vi "Documentation.vi"   [LabVIEW 2019, in "Inst.KH7008.lvlib" / "Inst.Krohn-Hite-7008.lvclass"]
uses:
  Inst.Krohn-Hite-7008.lvclass
  <vilib>/JKI/JKI SMO/SMO/SMO.lvclass
  Typedefs/Inst.Krohn-Hite-7008.getAll--Cluster.ctl
  Typedefs/Inst.Krohn-Hite-7008.device--Cluster.ctl
  Inst UI.Krohn-Hite-7008/Inst UI.Krohn-Hite-7008.lvclass
  Inst UI.Krohn-Hite-7008/Inst UI.Krohn-Hite-7008.UI--Cluster.ctl
  <userlib>/LevyLab/Instrument Framework/Instrument UI/Instrument UI.lvclass
  C:/Program Files (x86)/National Instruments/LabVIEW 2019/user.lib/LevyLab/Instrument Framework/Instrument Types/Amplifier/Instrument.Amplifier.lvclass
  C:/Program Files (x86)/National Instruments/LabVIEW 2019/user.lib/LevyLab/Instrument Framework/Instrument/Instrument.lvclass
  C:/Program Files (x86)/National Instruments/LabVIEW 2019/vi.lib/JKI/JKI SMO/SMO/SMO.lvclass
  Typedefs/Inst.Krohn-Hite-7008.Commands--Enum.ctl
  <userlib>/LevyLab/Instrument Framework/Instrument/Instrument.lvclass
  KH7008/typedefs/Input--Enum.ctl
  KH7008/KH7008.lvlib
  KH7008/typedefs/couple--Enum.ctl
  KH7008/typedefs/shunt--enum.ctl
  KH7008/typedefs/Filter--Enum.ctl
  KH7008/typedefs/gain--enum.ctl
  KH7008/typedefs/channel--numeric.ctl
  KH7008/typedefs/channelProperties--Cluster.ctl
  KH7008/typedefs/allChannelProperties--Array.ctl
  Typedefs/setAllChannelsRequest--Cluster.ctl
  C:/Program Files (x86)/National Instruments/LabVIEW 2019/user.lib/LevyLab/Instrument Framework/Instrument UI/Instrument UI.lvclass
  C:/Program Files (x86)/National Instruments/LabVIEW 2019/vi.lib/JKI/JKI SMO/SMO.UI/SMO.UI.lvclass
  <vilib>/JKI/JKI SMO/SMO.UI/SMO.UI.lvclass
  <userlib>/LevyLab/RemoteControl/RemoteControl/RemoteControl.lvclass
  <userlib>/LevyLab/Instrument Framework/Instrument/API/Instrument.sendMessageToProcess (string).vi
types:
  T1 = typedef "Inst.KH7008.lvlib/Inst.Krohn-Hite-7008.lvclass/Inst.Krohn-Hite-7008.device--Cluster.ctl" = cluster{"model":string, "device_id":string}
  T2 = typedef "Inst.KH7008.lvlib/Inst.Krohn-Hite-7008.lvclass/Inst.Krohn-Hite-7008.getAll--Cluster.ctl" = cluster{"allChannelProperties":T3}
  T3 = typedef "KH7008.lvlib/allChannelProperties--Array.ctl" = T4[]
  T4 = typedef "KH7008.lvlib/channelProperties--Cluster.ctl" = cluster{"channel":T5, "gain":T6, "input":T7, "shunt":T8, "couple":T9, "filter":T10}
  T5 = typedef "KH7008.lvlib/channel--numeric.ctl" = u16
  T6 = typedef "KH7008.lvlib/gain--enum.ctl" = enum16{"1", "10", "100", "1000"}
  T7 = typedef "KH7008.lvlib/Input--Enum.ctl" = enum16{"OFF", "SE+", "SE-", "DIFF"}
  T8 = typedef "KH7008.lvlib/shunt--enum.ctl" = enum16{"Open", "50", "500", "5k", "50k", "10M"}
  T9 = typedef "KH7008.lvlib/couple--Enum.ctl" = enum16{"AC", "DC"}
  T10 = typedef "KH7008.lvlib/Filter--Enum.ctl" = enum16{"OFF", "ON"}
  T11 = typedef "Inst.KH7008.lvlib/Inst.Krohn-Hite-7008.lvclass/Inst.Krohn-Hite-7008.Commands--Enum.ctl" = enum16{"getChannel", "getAllChannels", "setChannel", "setAllChannels"}
  T12 = typedef "Inst.KH7008.lvlib/Inst UI.Krohn-Hite-7008.lvclass/Inst UI.Krohn-Hite-7008.UI--Cluster.ctl" = cluster{"setAllChannelsRequest":T13}
  T13 = typedef "Inst.KH7008.lvlib/Inst.Krohn-Hite-7008.lvclass/setAllChannelsRequest--Cluster.ctl" = cluster{"allChannelProperties":T3}
  T14 = typedef "Instrument.lvlib/Instrument.lvclass/PublicEvents--Cluster.ctl" = cluster{"MessageFromProcess":refnum<user-event>}
  T15 = typedef "Instrument.lvlib/Instrument.lvclass/PrivateEvents--Cluster.ctl" = cluster{"MessageToProcess":refnum<user-event>, "LogData":refnum<user-event>, "LogDataMultiline":refnum<user-event>}
  T16 = typedef "Inst.KH7008.lvlib/Inst.Krohn-Hite-7008.lvclass/PublicEvents--Cluster.ctl" = cluster{"MessageFromProcess":refnum<user-event>}
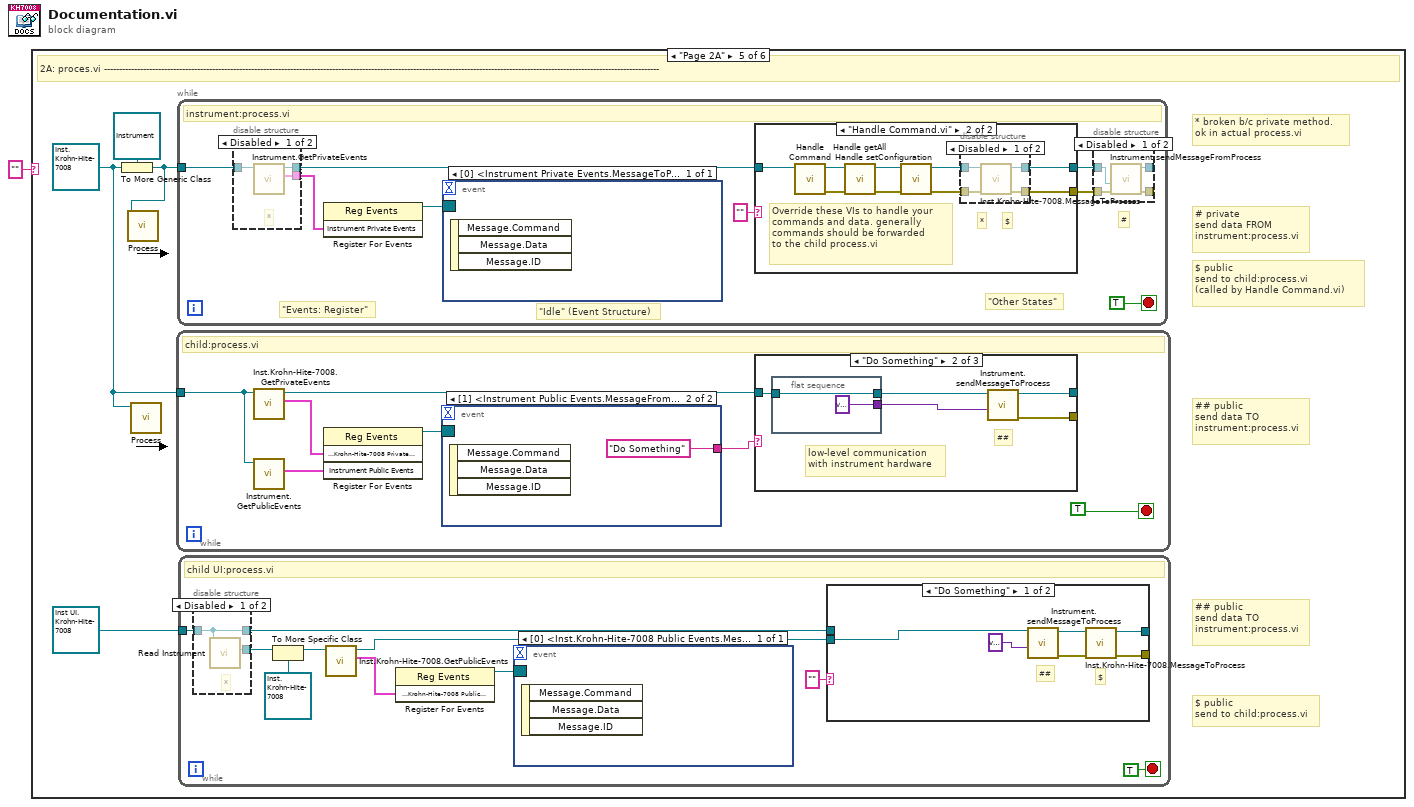
[diagram p0: block diagram]
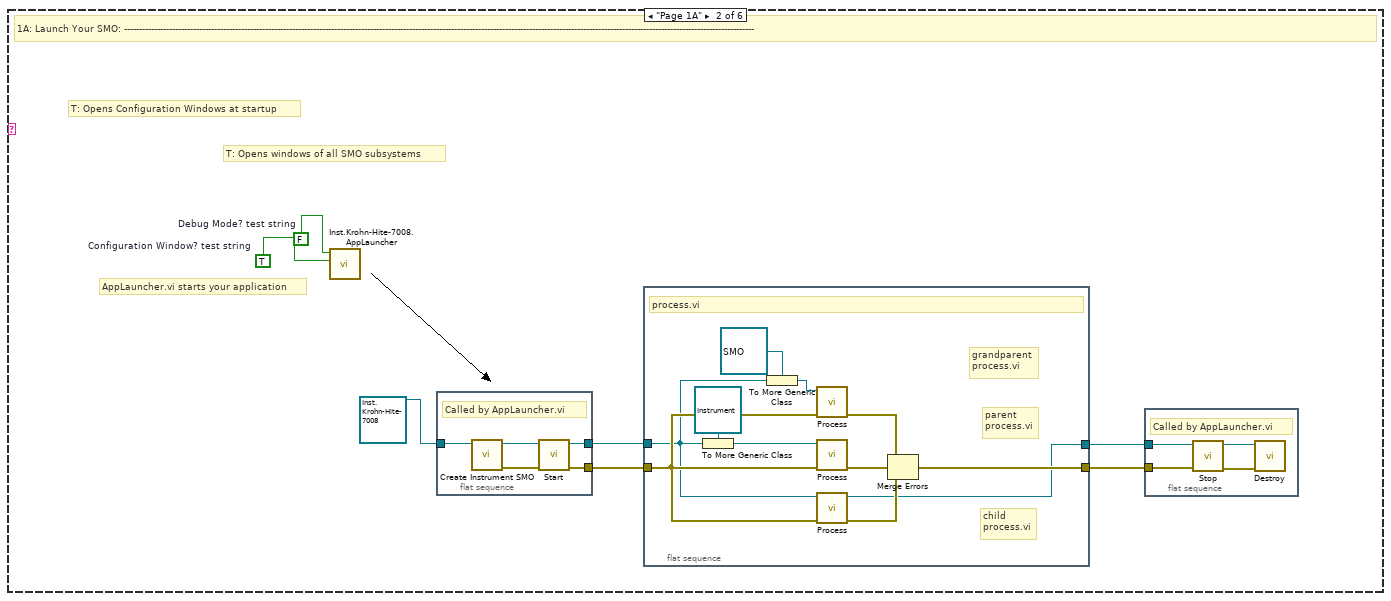
[diagram p3: hidden frame]
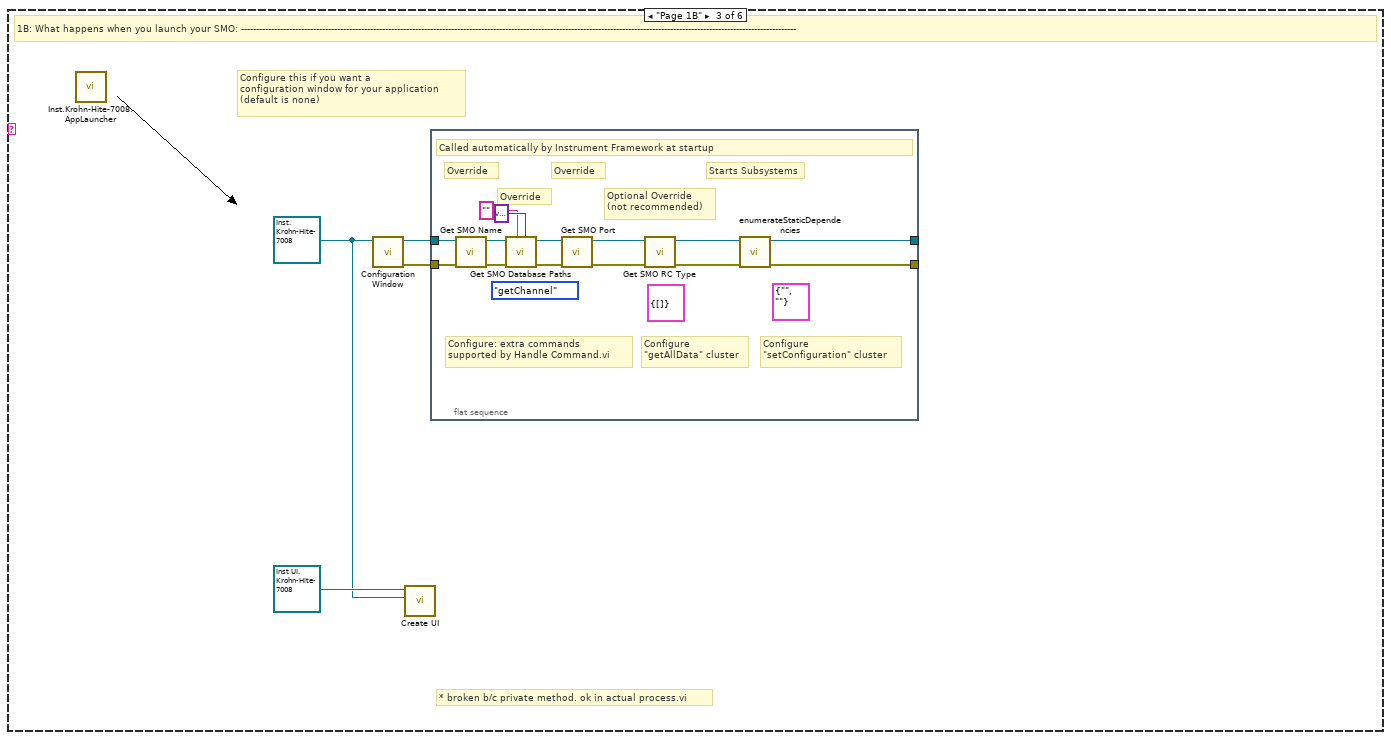
[diagram p4: hidden frame]
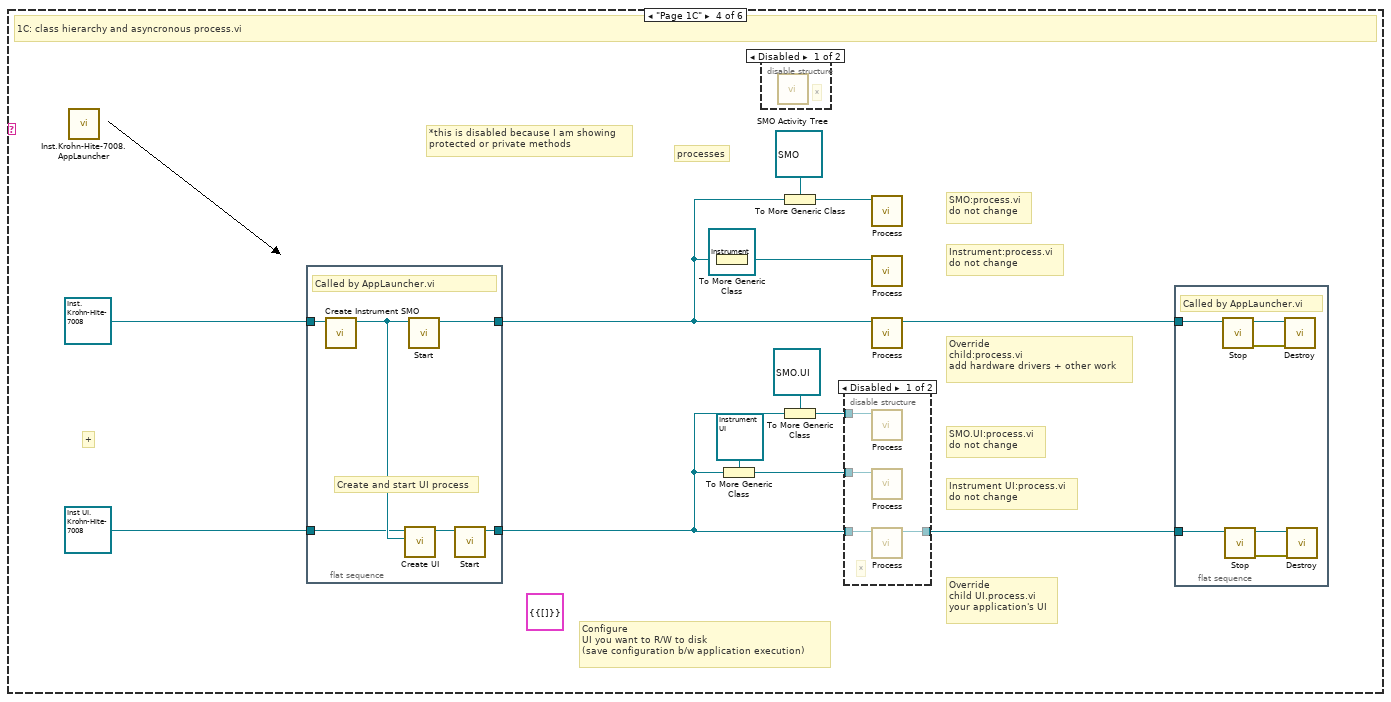
[diagram p5: hidden frame]
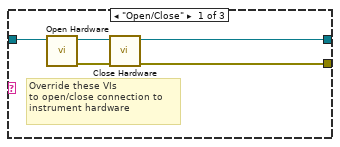
[diagram p10: hidden frame]
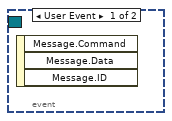
[diagram p12: hidden frame]
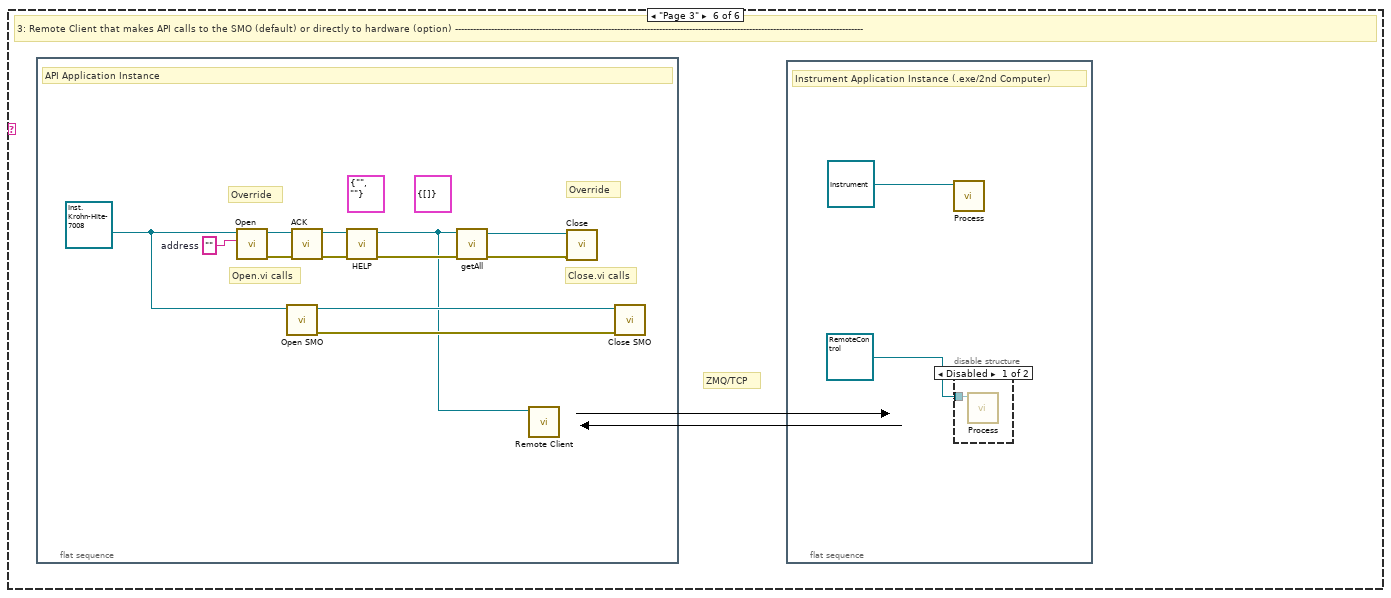
[diagram p17: hidden frame]
diagram:
  n1 = case shown="\"Page 2A\"" "" {
    frame Default {
    }
    frame "Page 1A" {
      w7 = TRUE  # Configuration Window? test string
      w8 = FALSE  # Debug Mode? test string
      # "AppLauncher.vi starts your application"
      # "T: Opens windows of all SMO subsystems"
      # "T: Opens Configuration Windows at startup"
      # "1A: Launch Your SMO: ------------------------------------------------------------------------------------------------------------------------------------------------------------------------------------------------------------------"
      n2 = call "Inst.Krohn-Hite-7008.AppLauncher.vi"("Config Window"=w7, "Debug Mode"=w8) -> ()  [unwired: 9 in, 1 out]
      n3 = flat-sequence {
        tunnel: [w26] -> w3
        tunnel: [w25] -> w5
        tunnel: refnum<class "Inst.Krohn-Hite-7008.lvclass"> refnum ("Instrument.Template.lvclass") -> [w24]
        frame #0 {
          # "Called by AppLauncher.vi"
          n4 = call <userlib>:"Create Instrument SMO.vi"("Instrument in"=w24) -> ("error out"=w27:errorcluster, "Instrument out"=w28:refnum<class "Inst.Krohn-Hite-7008.lvclass">)  [unwired: 9 in]
          n5 = call <vilib>:"Start.vi"("error in (no error)"=w27, "SMO"=w28) -> ("error out"=w25:errorcluster, "SMO out"=w26:refnum<class "Inst.Krohn-Hite-7008.lvclass">)  [unwired: 8 in]
        }
      }
      n6 = flat-sequence {
        tunnel: [w19] -> w6
        tunnel: w5 -> [w17]
        tunnel: [w11] -> w4
        tunnel: w3 -> [w10]
        frame #0 {
          # "child\nprocess.vi"
          # "grandparent\nprocess.vi"
          # "parent\nprocess.vi"
          # "process.vi"
          n7 = To More Generic Class(target class=refnum<class "Instrument.lvclass"> refnum ("Instrument"), reference=w10) -> (generic class reference=w16:refnum<class "Instrument.lvclass">)
          n8 = To More Generic Class(target class=refnum<class "SMO.lvclass"> refnum ("SMO"), reference=w10) -> (generic class reference=w18:refnum<class "SMO.lvclass">)
          n9 = call-dynamic "Process.vi"("error in"=w17, "SMO"=w18) -> ("error out"=w12:errorcluster)  [unwired: 8 in, 1 out]
          n10 = call-dynamic "Process.vi"("error in"=w17, "Instrument"=w16) -> ("error out"=w14:errorcluster)  [unwired: 8 in, 1 out]
          n11 = call-dynamic "Process.vi"("error in"=w17, "Inst.Krohn-Hite-7008"=w10) -> ("error out"=w13:errorcluster, "Inst.Krohn-Hite-7008 out"=w11:refnum<class "Inst.Krohn-Hite-7008.lvclass">)  [unwired: 8 in]
          n12 = Merge Errors(w12, w14, w13) -> (w19:errorcluster)
        }
      }
      n13 = flat-sequence {
        tunnel: w4 -> [w21]
        tunnel: w6 -> [w20]
        frame #0 {
          # "Called by AppLauncher.vi"
          n14 = call <vilib>:"Stop.vi"("error in (no error)"=w20, "SMO"=w21) -> ("error out"=w23:errorcluster, "SMO out"=w22:refnum<class "Inst.Krohn-Hite-7008.lvclass">)  [unwired: 8 in]
          n15 = call <vilib>:"Destroy.vi"("error in (no error)"=w23, "SMO"=w22) -> ()  [unwired: 9 in, 1 out]
        }
      }
    }
    frame "Page 1B" {
      w29 = refnum<class "Inst.Krohn-Hite-7008.lvclass"> refnum ("Instrument.Template.lvclass")
      # "* broken b/c private method. ok in actual process.vi"
      # "Configure this if you want a\nconfiguration window for your application\n(default is none)"
      # "1B: What happens when you launch your SMO: -----------------------------------------------------------------------------------------------------------------------------------------------------------------------------------------"
      n16 = call "Inst.Krohn-Hite-7008.AppLauncher.vi"() -> ()  [unwired: 11 in, 1 out]
      n17 = call-dynamic "Configuration Window.vi"("Inst.Krohn-Hite-7008 in"=w29) -> ("error out"=w31:errorcluster, "Inst.Krohn-Hite-7008 out"=w32:refnum<class "Inst.Krohn-Hite-7008.lvclass">)  [unwired: 9 in]
      n18 = call <userlib>:"Create UI.vi"("Instrument in"=w29, "Instrument UI"=refnum<class "Inst UI.Krohn-Hite-7008.lvclass"> refnum ("Instrument UI.Template.lvclass")) -> ()  [unwired: 8 in, 2 out]
      n19 = flat-sequence {
        tunnel: w32 -> [w42]
        tunnel: w31 -> [w37]
        tunnel: [w36] -> _
        tunnel: [w35] -> _
        frame #0 {
          (unwired) T1 {"model"="", "device_id"=""} ("Configuration")
          (unwired) T2 {"allChannelProperties"=[]} ("getAll")
          (unwired) Inst.Krohn-Hite-7008.Commands--Enum."getChannel" ("Commands")
          # "Configure\n\"setConfiguration\" cluster"
          # "Configure\n\"getAllData\" cluster"
          # "Configure: extra commands\nsupported by Handle Command.vi"
          # "Starts Subsystems"
          # "Override"
          # "Override"
          # "Override"
          # "Optional Override\n(not recommended)"
          # "Called automatically by Instrument Framework at startup"
          n20 = call-dynamic "Get SMO Name.vi"("error in (no error)"=w37, "Inst.Krohn-Hite-7008 in"=w42) -> ("error out"=w40:errorcluster, "Inst.Krohn-Hite-7008 out"=w41:refnum<class "Inst.Krohn-Hite-7008.lvclass">)  [unwired: 7 in, 1 out]
          n21 = call-dynamic "Get SMO Database Paths.vi"("getAll Cluster"=variant, "Paths"="" ("Default Paths"), "error in (no error)"=w40, "Inst.Krohn-Hite-7008 in"=w41) -> ("error out"=w38:errorcluster, "Inst.Krohn-Hite-7008 out"=w39:refnum<class "Inst.Krohn-Hite-7008.lvclass">)  [unwired: 5 in, 1 out]
          n22 = call-dynamic "Get SMO Port.vi"("error in (no error)"=w38, "Inst.Krohn-Hite-7008Instrument in"=w39) -> ("error out"=w43:errorcluster, "Inst.Krohn-Hite-7008Instrument out"=w44:refnum<class "Inst.Krohn-Hite-7008.lvclass">)  [unwired: 7 in, 1 out]
          n23 = call-dynamic "Get SMO RC Type.vi"("error in (no error)"=w43, "Instrument in"=w44) -> ("error out"=w45:errorcluster, "Instrument out"=w46:refnum<class "Inst.Krohn-Hite-7008.lvclass">)  [unwired: 7 in, 1 out]
          n24 = call-dynamic "enumerateStaticDependencies.vi"("error in (no error)"=w45, "Instrument"=w46) -> ("error out"=w36:errorcluster, "Instrument out"=w35:refnum<class "Inst.Krohn-Hite-7008.lvclass">)  [unwired: 7 in, 1 out]
        }
      }
    }
    frame "Page 1C" {
      (unwired) T12 {"setAllChannelsRequest"={"allChannelProperties"=[]}} ("UI")
      # "processes"
      # "SMO.UI:process.vi\ndo not change"
      # "Instrument UI:process.vi\ndo not change"
      # "Override\nchild:process.vi\nadd hardware drivers + other work"
      # "SMO:process.vi\ndo not change"
      # "Instrument:process.vi\ndo not change"
      # "*this is disabled because I am showing\nprotected or private methods"
      # "Configure\nUI you want to R/W to disk\n(save configuration b/w application execution)"
      # "Override\nchild UI.process.vi\nyour application's UI"
      # "+"
      # "1C: class hierarchy and asyncronous process.vi"
      n25 = call "Inst.Krohn-Hite-7008.AppLauncher.vi"() -> ()  [unwired: 11 in, 1 out]
      n26 = flat-sequence {
        tunnel: [w76] -> w59
        tunnel: refnum<class "Inst.Krohn-Hite-7008.lvclass"> refnum ("Instrument.Template.lvclass") -> [w75]
        tunnel: refnum<class "Inst UI.Krohn-Hite-7008.lvclass"> refnum ("Instrument UI.Template.lvclass") -> [w73]
        tunnel: [w71] -> w57
        frame #0 {
          # "Create and start UI process"
          # "Called by AppLauncher.vi"
          n27 = call <userlib>:"Create Instrument SMO.vi"("Instrument in"=w75) -> ("Instrument out"=w74:refnum<class "Inst.Krohn-Hite-7008.lvclass">)  [unwired: 9 in, 1 out]
          n28 = call <userlib>:"Create UI.vi"("Instrument in"=w74, "Instrument UI"=w73) -> ("Instrument UI out"=w72:refnum<class "Inst UI.Krohn-Hite-7008.lvclass">)  [unwired: 8 in, 1 out]
          n29 = call <vilib>:"Start.vi"("SMO"=w74) -> ("SMO out"=w76:refnum<class "Inst.Krohn-Hite-7008.lvclass">)  [unwired: 9 in, 1 out]
          n30 = call <vilib>:"Start.vi"("SMO"=w72) -> ("SMO out"=w71:refnum<class "Inst UI.Krohn-Hite-7008.lvclass">)  [unwired: 9 in, 1 out]
        }
      }
      n31 = To More Generic Class(target class=refnum<class "Instrument.lvclass"> refnum ("Instrument"), reference=w59) -> (generic class reference=w54:refnum<class "Instrument.lvclass">)
      n32 = To More Generic Class(target class=refnum<class "Instrument UI.lvclass"> refnum ("Instrument UI"), reference=w57) -> (generic class reference=w50:refnum<class "Instrument UI.lvclass">)
      n33 = disable-structure shown="Disabled" {
        frame Disabled {
          # "*"
          n34 = call <vilib>:"SMO Activity Tree.vi"() -> ()  [unwired: 12 in]
        }
        frame Enabled {
        }
      }
      n35 = To More Generic Class(target class=refnum<class "SMO.lvclass"> refnum ("SMO"), reference=w59) -> (generic class reference=w55:refnum<class "SMO.lvclass">)
      n36 = To More Generic Class(target class=refnum<class "SMO.UI.lvclass"> refnum ("SMO.UI"), reference=w57) -> (generic class reference=w48:refnum<class "SMO.UI.lvclass">)
      n37 = disable-structure shown="Disabled" {
        disable-tunnel: w57 -> [w64 _]
        disable-tunnel: [w63 _] -> w56
        disable-tunnel: w50 -> [w62 _]
        disable-tunnel: w48 -> [w61 _]
        frame Disabled {
          # "*"
          n38 = call-dynamic "Process.vi"("SMO.UI"=w61) -> ()  [unwired: 9 in, 2 out]
          n39 = call-dynamic "Process.vi"("Instrument UI in"=w62) -> ()  [unwired: 9 in, 2 out]
          n40 = call-dynamic "Process.vi"("Inst UI.Krohn-Hite-7008"=w64) -> ("Inst UI.Krohn-Hite-7008 out"=w63:refnum<class "Inst UI.Krohn-Hite-7008.lvclass">)  [unwired: 9 in, 1 out]
        }
        frame Enabled {
        }
      }
      n41 = call-dynamic "Process.vi"("SMO"=w55) -> ()  [unwired: 9 in, 2 out]
      n42 = call-dynamic "Process.vi"("Instrument"=w54) -> ()  [unwired: 9 in, 2 out]
      n43 = call-dynamic "Process.vi"("Inst.Krohn-Hite-7008"=w59) -> ("Inst.Krohn-Hite-7008 out"=w60:refnum<class "Inst.Krohn-Hite-7008.lvclass">)  [unwired: 9 in, 1 out]
      n44 = flat-sequence {
        tunnel: w60 -> [w68]
        tunnel: w56 -> [w66]
        frame #0 {
          # "Called by AppLauncher.vi"
          n45 = call <vilib>:"Stop.vi"("SMO"=w68) -> ("error out"=w70:errorcluster, "SMO out"=w69:refnum<class "Inst.Krohn-Hite-7008.lvclass">)  [unwired: 9 in]
          n46 = call <vilib>:"Stop.vi"("SMO"=w66) -> ("error out"=w67:errorcluster, "SMO out"=w65:refnum<class "Inst UI.Krohn-Hite-7008.lvclass">)  [unwired: 9 in]
          n47 = call <vilib>:"Destroy.vi"("error in (no error)"=w70, "SMO"=w69) -> ()  [unwired: 9 in, 1 out]
          n48 = call <vilib>:"Destroy.vi"("error in (no error)"=w67, "SMO"=w65) -> ()  [unwired: 9 in, 1 out]
        }
      }
    }
    frame "Page 2A" {
      w77 = refnum<class "Inst.Krohn-Hite-7008.lvclass"> refnum ("Instrument.Template.lvclass")
      # "## public\nsend data TO\ninstrument:process.vi"
      # "$ public\nsend to child:process.vi"
      # "## public\nsend data TO\ninstrument:process.vi"
      # "$ public\nsend to child:process.vi\n(called by Handle Command.vi)"
      # "# private\nsend data FROM\ninstrument:process.vi"
      # "* broken b/c private method.\nok in actual process.vi"
      # "2A: proces.vi -----------------------------------------------------------------------------------------------------------------------------------------------------------------------------------------"
      n49 = To More Generic Class(target class=refnum<class "Instrument.lvclass"> refnum ("Instrument"), reference=w77) -> (generic class reference=w78:refnum<class "Instrument.lvclass">)
      n50 = call-dynamic "Process.vi"("Instrument"=w78) -> ()  [unwired: 9 in, 2 out]
      n51 = call-dynamic "Process.vi"("Inst.Krohn-Hite-7008"=w77) -> ()  [unwired: 9 in, 2 out]
      n52 = while {
        tunnel: w77 -> [w103]
        stop <- TRUE stop-if-true
        # "child:process.vi"
        n53 = call "Inst.Krohn-Hite-7008.GetPrivateEvents.vi"("Inst.Krohn-Hite-7008 in"=w103) -> ("Inst.Krohn-Hite-7008 Private Events"=w107:cluster{"MessageToProcess":refnum<user-event>}, "Inst.Krohn-Hite-7008 out"=w105:refnum<class "Inst.Krohn-Hite-7008.lvclass">)  [unwired: 8 in, 1 out]
        n54 = call <userlib>:"Instrument.GetPublicEvents.vi"("Instrument"=w103) -> ("Instrument Public Events"=w104:T14)  [unwired: 8 in, 2 out]
        n55 = register-events(w107, w104) -> (reference out=w106:refnum<event-registration>)  [unwired: 2 in, 1 out]
        n56 = event shown="[1] <Instrument Public Events.MessageFromProcess>: User Event" {
          selector: w106 -> [_ _]
          dyn-events: _ -> [_ _]
          timeout: _ -> [_ _]
          tunnel: [_ "Do Something"] -> w101
          event User Event {
            n57 = event-data() -> ()  [unwired: 1 in, 3 out]
          }
          event User Event {
            n58 = event-data() -> ()  [unwired: 1 in, 3 out]
          }
        }
        n59 = case shown="\"Do Something\"" w101 {
          tunnel: w105 -> [w110 w115 w120]
          tunnel: [w109 w117 w120] -> _
          tunnel: [w108 w116 _] -> _
          frame "Open/Close" {
            # "Override these VIs\nto open/close connection to\ninstrument hardware"
            n60 = call-dynamic "Open Hardware.vi"("Inst.Krohn-Hite-7008 in"=w110) -> ("error out"=w112:errorcluster, "Inst.Krohn-Hite-7008 out"=w111:refnum<class "Inst.Krohn-Hite-7008.lvclass">)  [unwired: 9 in]
            n61 = call-dynamic "Close Hardware.vi"("error in (no error)"=w112, "Inst.Krohn-Hite-7008 in"=w111) -> ("error out"=w108:errorcluster, "Inst.Krohn-Hite-7008 out"=w109:refnum<class "Inst.Krohn-Hite-7008.lvclass">)  [unwired: 8 in]
          }
          frame "Do Something" {
            # "##"
            # "low-level communication\nwith instrument hardware"
            n62 = flat-sequence {
              tunnel: w115 -> [w119]
              tunnel: [w119] -> w114
              tunnel: [variant ("Data")] -> w113
              frame #0 {
              }
            }
            n63 = call-poly <userlib>:"Instrument.sendMessageToProcess.vi"("Data"=w113, "Instrument"=w114) -> ("error out"=w116:errorcluster, "Instrument out"=w117:refnum<class "Inst.Krohn-Hite-7008.lvclass">)  [unwired: 8 in]
          }
          frame Default {
          }
        }
      }
      n64 = while {
        tunnel: w78 -> [w128]
        stop <- TRUE stop-if-true
        # "#"
        # "\"Other States\""
        # "\"Idle\" (Event Structure)"
        # "\"Events: Register\""
        # "instrument:process.vi"
        n65 = disable-structure shown="Disabled" {
          disable-tunnel: w128 -> [w152 w153]
          disable-tunnel: [w151 w153] -> w127
          disable-tunnel: [w150 _] -> w126
          frame Disabled {
            # "*"
            n66 = call <userlib>:"Instrument.GetPrivateEvents.vi"("Instrument"=w152) -> ("Instrument Private Events"=w150:T15, "Instrument out"=w151:refnum<class "Instrument.lvclass">)  [unwired: 8 in, 1 out]
          }
          frame Enabled {
          }
        }
        n67 = register-events(w126) -> (reference out=w125:refnum<event-registration>)  [unwired: 2 in, 1 out]
        n68 = event shown="[0] <Instrument Private Events.MessageToProcess>: User Event" {
          selector: w125 -> [_]
          dyn-events: _ -> [_]
          timeout: _ -> [_]
          event User Event {
            n69 = event-data() -> ()  [unwired: 1 in, 3 out]
          }
        }
        n70 = case shown="\"Handle Command.vi\"" "" {
          tunnel: w127 -> [w134 w143]
          tunnel: [w134 w137] -> w124
          tunnel: [_ w136] -> w123
          frame Default {
          }
          frame "Handle Command.vi" {
            # "*"
            # "$"
            # "Override these VIs to handle your\ncommands and data. generally \ncommands should be forwarded\nto the child process.vi"
            n71 = call-dynamic "Handle Command.vi"("Instrument in"=w143) -> ("error out"=w139:errorcluster, "Instrument out"=w142:refnum<class "Instrument.lvclass">)  [unwired: 7 in, 2 out]
            n72 = call-dynamic "Handle getAll.vi"("error in (no error)"=w139, "Instrument in"=w142) -> ("error out"=w140:errorcluster, "Instrument out"=w141:refnum<class "Instrument.lvclass">)  [unwired: 7 in, 1 out]
            n73 = call-dynamic "Handle setConfiguration.vi"("error in (no error)"=w140, "Instrument in"=w141) -> ("error out"=w135:errorcluster, "Instrument out"=w138:refnum<class "Instrument.lvclass">)  [unwired: 8 in]
            n74 = disable-structure shown="Disabled" {
              disable-tunnel: w138 -> [w147 w149]
              disable-tunnel: [w146 w149] -> w137
              disable-tunnel: [w145 w148] -> w136
              disable-tunnel: w135 -> [w144 w148]
              frame Disabled {
                n75 = call "Inst.Krohn-Hite-7008.MessageToProcess.vi"("error in (no error)"=w144, "Inst.Krohn-Hite-7008 in"=w147) -> ("error out"=w145:errorcluster, "Inst.Krohn-Hite-7008 out"=w146:refnum<class "Inst.Krohn-Hite-7008.lvclass">)  [unwired: 8 in]
              }
              frame Enabled {
              }
            }
          }
        }
        n76 = disable-structure shown="Disabled" {
          disable-tunnel: w124 -> [w133 _]
          disable-tunnel: w123 -> [w132 _]
          disable-tunnel: [w131 _] -> _
          disable-tunnel: [w130 _] -> _
          frame Disabled {
            n77 = call <userlib>:"Instrument.sendMessageFromProcess.vi"("error in (no error)"=w132, "Data"=w133) -> ("error out"=w131:errorcluster, "Instrument out"=w130:refnum<class "Instrument.lvclass">)  [unwired: 8 in]
          }
          frame Enabled {
          }
        }
      }
      n78 = while {
        tunnel: refnum<class "Inst UI.Krohn-Hite-7008.lvclass"> refnum ("Instrument UI.Template.lvclass") -> [w89]
        stop <- TRUE stop-if-true
        # "child UI:process.vi"
        n79 = disable-structure shown="Disabled" {
          disable-tunnel: w89 -> [w98 w100]
          disable-tunnel: [w99 _] -> w87
          disable-tunnel: [w98 w100] -> w83
          frame Disabled {
            # "*"
            n80 = call <userlib>:"Read Instrument.vi"("Instrument UI in"=w98) -> ("Instrument"=w99:refnum<class "Instrument.lvclass">)  [unwired: 8 in, 2 out]
          }
          frame Enabled {
          }
        }
        n81 = To More Specific Class(target class=refnum<class "Inst.Krohn-Hite-7008.lvclass"> refnum ("Instrument.Template.lvclass"), reference=w87) -> (specific class reference=w86:refnum<class "Inst.Krohn-Hite-7008.lvclass">)  [unwired: 1 in, 1 out]
        n82 = call "Inst.Krohn-Hite-7008.GetPublicEvents.vi"("Inst.Krohn-Hite-7008 in"=w86) -> ("Inst.Krohn-Hite-7008 Public Events"=w84:T16, "Inst.Krohn-Hite-7008 out"=w82:refnum<class "Inst.Krohn-Hite-7008.lvclass">)  [unwired: 8 in, 1 out]
        n83 = register-events(w84) -> (reference out=w85:refnum<event-registration>)  [unwired: 2 in, 1 out]
        n84 = event shown="[0] <Inst.Krohn-Hite-7008 Public Events.MessageFromProcess>: User Event" {
          selector: w85 -> [_]
          dyn-events: _ -> [_]
          timeout: _ -> [_]
          event User Event {
            n85 = event-data() -> ()  [unwired: 1 in, 3 out]
          }
        }
        n86 = case shown="\"Do Something\"" "" {
          tunnel: w83 -> [_ _]
          tunnel: [w93 w97] -> _
          tunnel: [w92 _] -> _
          tunnel: w82 -> [w94 w97]
          frame "Do Something" {
            # "##"
            # "$"
            n87 = call-poly <userlib>:"Instrument.sendMessageToProcess.vi"("Data"=variant, "Instrument"=w94) -> ("error out"=w91:errorcluster, "Instrument out"=w95:refnum<class "Inst.Krohn-Hite-7008.lvclass">)  [unwired: 8 in]
            n88 = call "Inst.Krohn-Hite-7008.MessageToProcess.vi"("error in (no error)"=w91, "Inst.Krohn-Hite-7008 in"=w95) -> ("error out"=w92:errorcluster, "Inst.Krohn-Hite-7008 out"=w93:refnum<class "Inst.Krohn-Hite-7008.lvclass">)  [unwired: 8 in]
          }
          frame Default {
          }
        }
      }
    }
    frame "Page 3" {
      # "ZMQ/TCP"
      # "3: Remote Client that makes API calls to the SMO (default) or directly to hardware (option) ----------------------------------------------------------------------------------------------------------------------------------------"
      n89 = flat-sequence {
        frame #0 {
          w163 = ""  # address
          (unwired) T1 {"model"="", "device_id"=""} ("Configuration")
          (unwired) T2 {"allChannelProperties"=[]} ("getAll")
          w168 = refnum<class "Inst.Krohn-Hite-7008.lvclass"> refnum ("Instrument.Template.lvclass")
          # "Close.vi calls"
          # "Open.vi calls"
          # "Override"
          # "Override"
          # "API Application Instance"
          n90 = call-dynamic "Open.vi"("address"=w163, "Inst.Krohn-Hite-7008 in"=w168) -> ("error out"=w167:errorcluster, "Inst.Krohn-Hite-7008 out"=w166:refnum<class "Inst.Krohn-Hite-7008.lvclass">)  [unwired: 8 in]
          n91 = call <userlib>:"Open SMO.vi"("Instrument in"=w168) -> ("error out"=w161:errorcluster, "Instrument out"=w162:refnum<class "Inst.Krohn-Hite-7008.lvclass">)  [unwired: 9 in]
          n92 = call <userlib>:"ACK.vi"("error in (no error)"=w167, "Instrument in"=w166) -> ("error out"=w165:errorcluster, "Instrument out"=w164:refnum<class "Inst.Krohn-Hite-7008.lvclass">)  [unwired: 7 in, 1 out]
          n93 = call <userlib>:"HELP.vi"("error in (no error)"=w165, "Instrument in"=w164) -> ("error out"=w158:errorcluster, "Instrument in"=w157:refnum<class "Inst.Krohn-Hite-7008.lvclass">)  [unwired: 7 in, 1 out]
          n94 = call <userlib>:"getAll.vi"("error in (no error)"=w158, "Instrument in"=w157) -> ("error out"=w160:errorcluster, "Instrument out"=w159:refnum<class "Inst.Krohn-Hite-7008.lvclass">)  [unwired: 7 in, 1 out]
          n95 = call <userlib>:"Remote Client.vi"("Instrument in"=w157) -> ()  [unwired: 7 in, 4 out]
          n96 = call-dynamic "Close.vi"("error in (no error)"=w160, "Inst.Krohn-Hite-7008 in"=w159) -> ()  [unwired: 8 in, 2 out]
          n97 = call <userlib>:"Close SMO.vi"("error in (no error)"=w161, "Instrument in"=w162) -> ()  [unwired: 8 in, 2 out]
        }
      }
      n98 = flat-sequence {
        frame #0 {
          # "Instrument Application Instance (.exe/2nd Computer)"
          n99 = call-dynamic "Process.vi"("Instrument"=refnum<class "Instrument.lvclass"> refnum) -> ()  [unwired: 9 in, 2 out]
          n100 = disable-structure shown="Disabled" {
            disable-tunnel: refnum<class "RemoteControl.lvclass"> refnum ("RemoteControl out") -> [w156 _]
            frame Disabled {
              n101 = call-dynamic "Process.vi"("RemoteControl"=w156) -> ()  [unwired: 9 in, 2 out]
            }
            frame Enabled {
            }
          }
        }
      }
    }
  }
